vi "Initialize Page Number.vi"(8 "error in (no error)":errorcluster, 11 "Sensor Model in":refnum<class "Sensor Model.lvclass">) -> (0 "error out":errorcluster, 3 "Sensor Model out":refnum<class "Sensor Model.lvclass">)   [LabVIEW 2013, in "Sensor Model.lvlib" / "Sensor Model.lvclass"]
uses:
  Sensor Model.lvclass
  Sensor Model.lvclass/Sensor Model.ctl
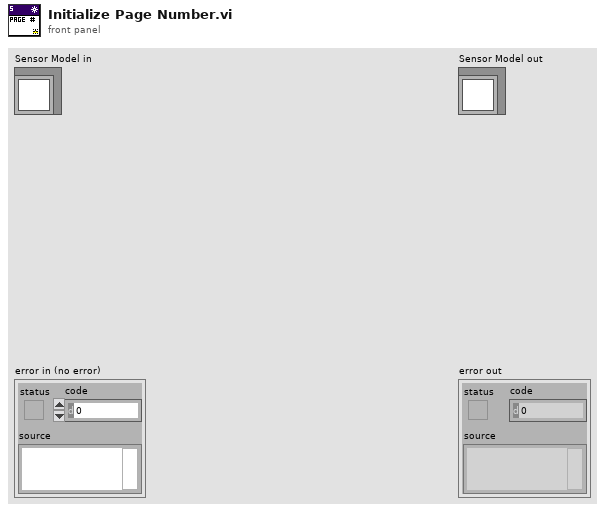
[diagram p1: front panel]
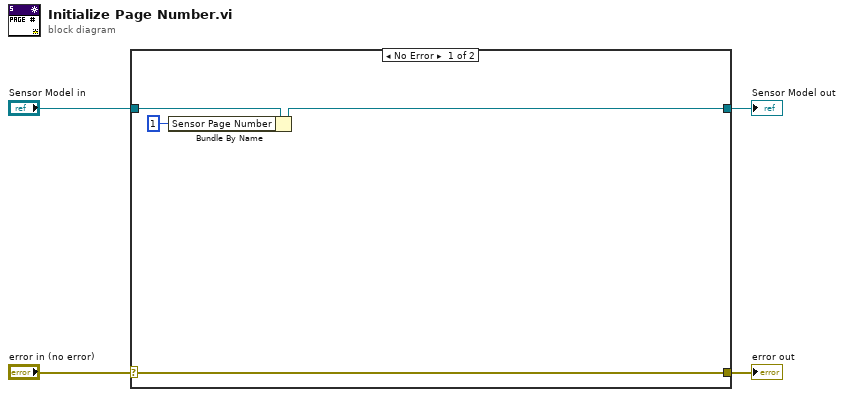
[diagram p0: block diagram]
diagram:
  n1 = case shown="No Error" "error in (no error)" {
    selector: "error in (no error)" -> [w7 w10]
    tunnel: [w7 w10] -> w3
    tunnel: [w6 w9] -> w1
    tunnel: "Sensor Model in" -> [w8 w9]
    frame No Error {
      n2 = Bundle By Name(cluster=w8, "Sensor Page Number"=1 ("Page Number")) -> (w6:refnum<class "Sensor Model.lvclass">)
    }
    frame Error {
    }
  }
  "error out" <- w3
  "Sensor Model out" <- w1
